vi "Keithley Temperature measurement improved.vi"() -> ()   [LabVIEW 2016]
doc: "This example VI shows how to use thermocouples to take a temperature measurement.\n\nNote:\nFor front panel measurements, make sure the Input switch is in the out position(F)\nFor plug-in card measurements, make sure the Input switch is in the in poisition(R)"
uses:
  Documents/keithley_27xx/Keithley 27XX/Public/Configure/Measurement Specific/Configure FRTD.vi
  Documents/keithley_27xx/Keithley 27XX/Public/Configure/Measurement Specific/Configure Thermocouple.vi
  Documents/keithley_27xx/Keithley 27XX/Public/Configure/Measurement Specific/Configure Thermistor.vi
  Documents/keithley_27xx/Keithley 27XX/Public/Data/Read Multiple Direct.vi
  Documents/keithley_27xx/Keithley 27XX/Keithley 27XX.lvlib
panel:
  in  "Sample Size":dbl
  in  "Sensor Type":string(combo)
  in  "Delta3":dbl=1.0
  in  "Beta3":dbl=0.1
  in  "Alpha3":dbl=0.0038
  in  "Delta2":dbl=1.0
  in  "Beta2":dbl=0.1
  in  "Alpha2":dbl=0.0038
  in  "Delta1":dbl=1.0
  in  "Beta1":dbl=0.1
  in  "Alpha1":dbl=0.0038
  in  "Serial Configuration":T1={"Baud Rate (9600)"=9600, "Flow Control (1: XON/XOFF)"=1, "Termination Char (0:CR)"=0} {"Termination Char (0:CR)" items=["CR", "LF", "CRLF (Do not use)", "LFCR (Do not use)"]; "Flow Control (1: XON/XOFF)" items=["None", "XON/XOFF", "RTS/CTS (2701 Only)", "XON/XOFF & RTS/CTS (2701 Only)"]; "Baud Rate (9600)" items=["300"=300, "600"=600, "1200"=1200, "2400"=2400, "4800"=4800, "9600"=9600, "19.2k"=19200, "38.4k (2701 Only)"=38400, "57.6k (2701 Only)"=57600, "115.2k (2701 Only)"=115200]}
  in  "VISA resource name":refnum<visa-resource-name>="TCPIP0::192.168.69.200::1394::SOCKET"
  out "Output3":dbl[](array[numeric])
  in  "Channel (101) 3":string="117"
  out "Output2":dbl[](array[numeric])
  in  "Channel (101) 2":string="114"
  in  "stop":bool
  out "Output1":dbl[](array[numeric])
  in  "Channel (101)":string="113"
  in  "Temperature (0: Celsius)":u16(ring) items=["Celsius", "Fahrenheit", "Kelvin"]
  # "*For front panel measurements, make sure the Input switch is in the out position(F)*\n  For plug-in card measurements, make sure the Input switch is in the in position(R)"
  # "© 2005 National Instruments Corporation.  ALL RIGHTS RESERVED."
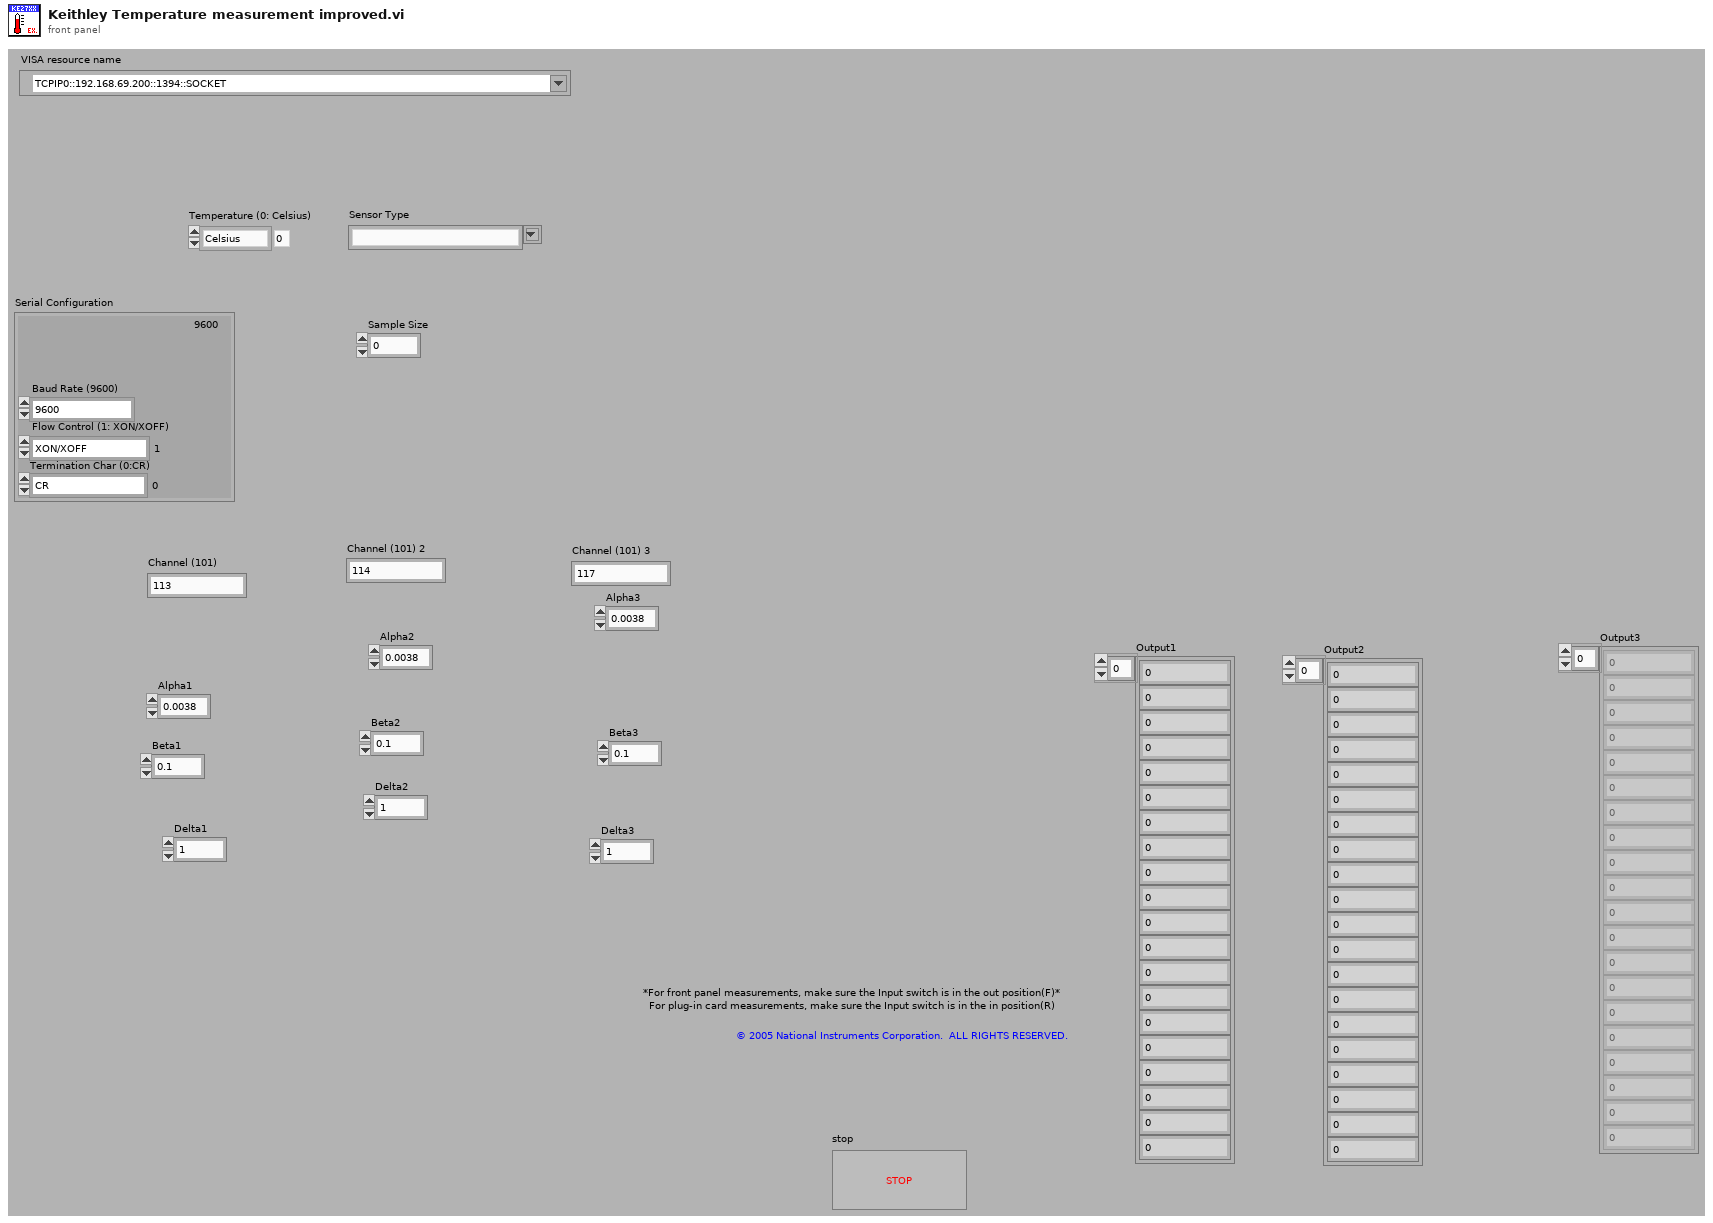
[diagram p1: front panel]
types:
  T1 = cluster{"Baud Rate (9600)":u32, "Flow Control (1: XON/XOFF)":u16, "Termination Char (0:CR)":u16}
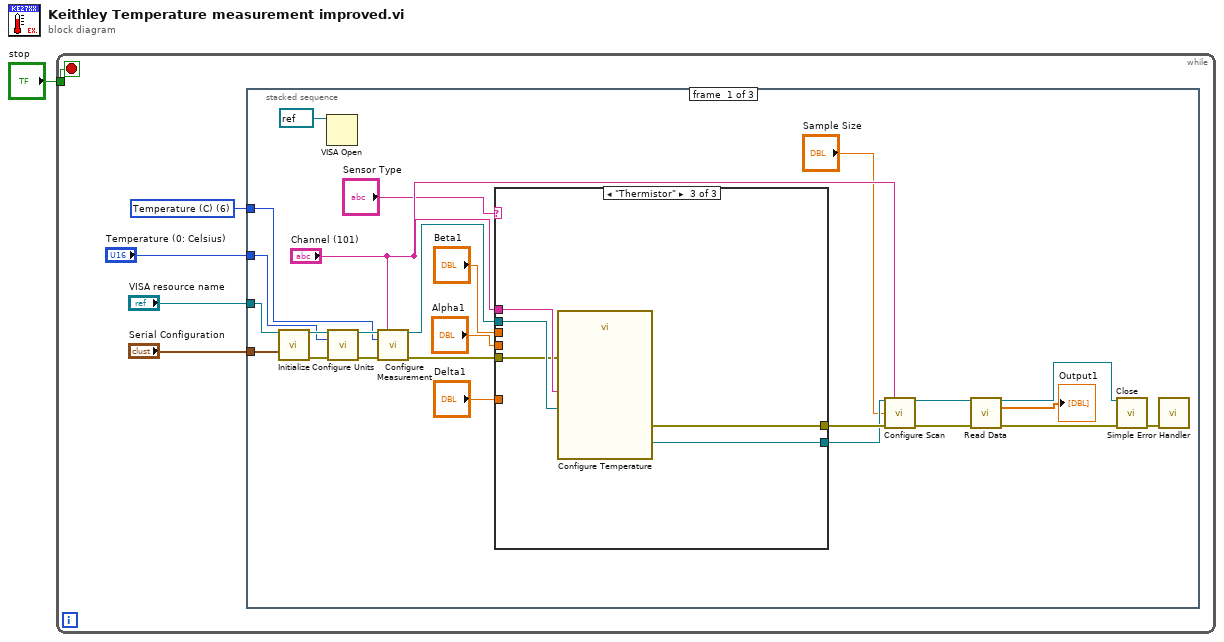
[diagram p0: block diagram]
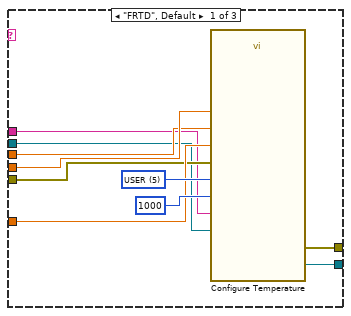
[diagram p2: hidden frame]
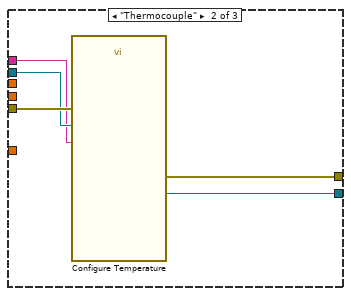
[diagram p3: hidden frame]
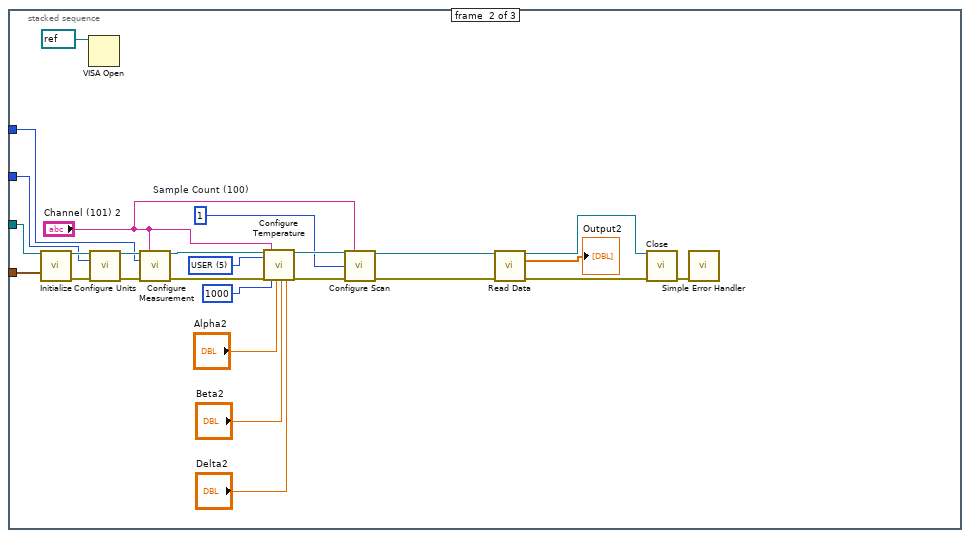
[diagram p4: hidden frame]
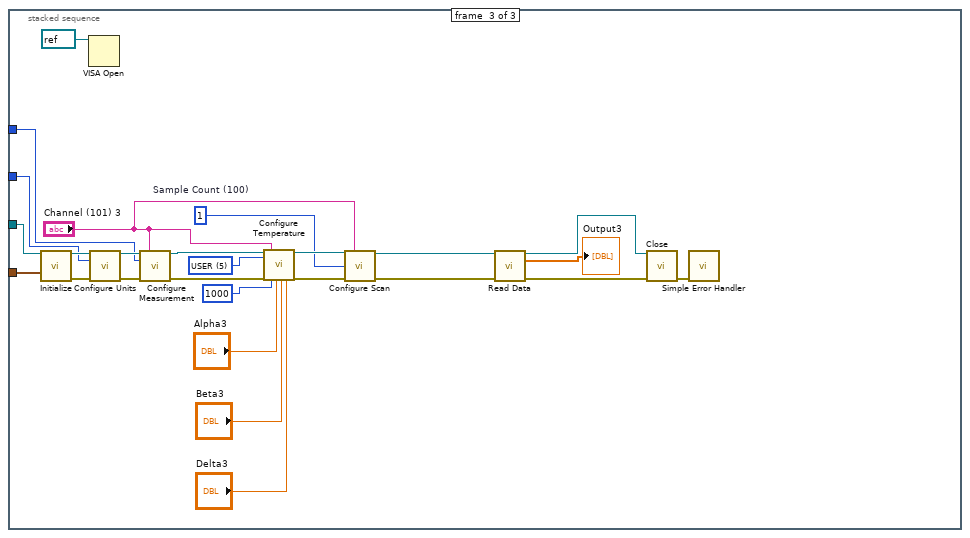
[diagram p5: hidden frame]
diagram:
  n1 = while {
    tunnel: "stop" -> [w2]
    stop <- w2 stop-if-true
    w4 = u16 6 items=["DC Voltage", "AC Voltage", "DC Current", "AC Current", "Resistance", "Four-Wire Resistance", "Temperature (C)", "Frequency", "Period", "Continuity"] ("Function (0: DC Voltage)")
    n2 = stacked-sequence {
      tunnel: "VISA resource name" -> [w20 w57 w84]
      tunnel: "Serial Configuration" -> [w19 w58 w83]
      tunnel: w4 -> [w18 w53 w79]
      tunnel: "Temperature (0: Celsius)" -> [w17 w52 w78]
      frame #0 {
        n3 = call "Initialize.vi"("VISA resource name"=w20, "Serial Configuration"=w19) -> ("VISA resource name out"=w30:refnum<visa-resource-name>, "error out"=w24:errorcluster)  [unwired: 12 in]
        n4 = VISA Open(VISA resource name=refnum<visa-resource-name> refnum) -> ()  [unwired: 4 in, 2 out]
        n5 = call "Configure Units.vi"("VISA resource name"=w30, "Temperature (0: Celsius)"=w17, "error in (no error)"=w24) -> ("VISA resource name out"=w31:refnum<visa-resource-name>, "error out"=w23:errorcluster)  [unwired: 11 in]
        n6 = call "Configure Measurement.vi"("VISA resource name"=w31, "Scan List (Empty)"="Channel (101)", "Function (0: DC Voltage)"=w18, "error in (no error)"=w23) -> ("VISA resource name out"=w10:refnum<visa-resource-name>, "error out"=w11:errorcluster)  [unwired: 10 in]
        n7 = case shown="\"Thermistor\"" "Sensor Type" {
          tunnel: [w40 w45 w51] -> w16
          tunnel: [w41 w46 w50] -> w15
          tunnel: "Delta1" -> [w35 _ _]
          tunnel: "Beta1" -> [w36 _ _]
          tunnel: "Alpha1" -> [w37 _ _]
          tunnel: w11 -> [w34 w44 w47]
          tunnel: w10 -> [w33 w43 w48]
          tunnel: "Channel (101)" -> [w32 w42 w49]
          frame "FRTD", Default {
            w39 = u16 5 items=["PT100", "D100", "F100", "PT3916", "PT385", "USER"] ("FRTD Type (0: PT100)")
            n8 = call-poly "Configure Temperature.vi"("VISA resource name"=w33, "FRTD Type (0: PT100)"=w39, "error in (no error)"=w34, "Scan List (Empty)"=w32, "R Zero (100)"=1000, "Alpha (0.00385)"=w37, "Beta (0.111)"=w36, "Delta (1.507)"=w35) -> ("VISA resource name out"=w41:refnum<visa-resource-name>, "error out"=w40:errorcluster)  [unwired: 10 in]
          }
          frame "Thermocouple" {
            n9 = call-poly "Configure Temperature.vi"("VISA resource name"=w43, "error in (no error)"=w44, "Scan List (Empty)"=w42) -> ("VISA resource name out"=w46:refnum<visa-resource-name>, "error out"=w45:errorcluster)  [unwired: 15 in]
          }
          frame "Thermistor" {
            n10 = call-poly "Configure Temperature.vi"("VISA resource name"=w48, "error in (no error)"=w47, "Scan List (Empty)"=w49) -> ("VISA resource name out"=w50:refnum<visa-resource-name>, "error out"=w51:errorcluster)  [unwired: 15 in]
          }
        }
        n11 = call "Configure Scan.vi"("VISA resource name"=w15, "Channel List (101:110)"="Channel (101)", "Sample Count (100)"="Sample Size", "error in (no error)"=w16) -> ("VISA resource name out"=w27:refnum<visa-resource-name>, "error out"=w28:errorcluster)  [unwired: 10 in]
        n12 = call-poly "Read Data.vi"("VISA resource name"=w27, "error in (no error)"=w28) -> ("VISA resource name out"=w25:refnum<visa-resource-name>, "Measurement Data"=→"Output1":dbl[], "error out"=w26:errorcluster)  [unwired: 8 in, 3 out]
        n13 = call "Close.vi"("VISA resource name"=w25, "error in (no error)"=w26) -> ("error out"=w29:errorcluster)  [unwired: 13 in]
        n14 = call <vilib>:"Simple Error Handler.vi"("error in (no error)"=w29) -> ()  [unwired: 4 in, 5 out]
      }
      frame #1 {
        w62 = u16 5 items=["PT100", "D100", "F100", "PT3916", "PT385", "USER"] ("FRTD Type (0: PT100)")
        w64 = 1  # Sample Count (100)
        n15 = call "Initialize.vi"("VISA resource name"=w57, "Serial Configuration"=w58) -> ("VISA resource name out"=w75:refnum<visa-resource-name>, "error out"=w67:errorcluster)  [unwired: 12 in]
        n16 = VISA Open(VISA resource name=refnum<visa-resource-name> refnum) -> ()  [unwired: 4 in, 2 out]
        n17 = call "Configure Units.vi"("VISA resource name"=w75, "Temperature (0: Celsius)"=w52, "error in (no error)"=w67) -> ("VISA resource name out"=w76:refnum<visa-resource-name>, "error out"=w66:errorcluster)  [unwired: 11 in]
        n18 = call "Configure Measurement.vi"("VISA resource name"=w76, "Scan List (Empty)"="Channel (101) 2", "Function (0: DC Voltage)"=w53, "error in (no error)"=w66) -> ("VISA resource name out"=w65:refnum<visa-resource-name>, "error out"=w77:errorcluster)  [unwired: 10 in]
        n19 = call-poly "Configure Temperature.vi"("VISA resource name"=w65, "FRTD Type (0: PT100)"=w62, "error in (no error)"=w77, "Scan List (Empty)"="Channel (101) 2", "R Zero (100)"=1000, "Alpha (0.00385)"="Alpha2", "Beta (0.111)"="Beta2", "Delta (1.507)"="Delta2") -> ("VISA resource name out"=w73:refnum<visa-resource-name>, "error out"=w72:errorcluster)  [unwired: 10 in]
        n20 = call "Configure Scan.vi"("VISA resource name"=w73, "Channel List (101:110)"="Channel (101) 2", "Sample Count (100)"=w64, "error in (no error)"=w72) -> ("VISA resource name out"=w70:refnum<visa-resource-name>, "error out"=w71:errorcluster)  [unwired: 10 in]
        n21 = call-poly "Read Data.vi"("VISA resource name"=w70, "error in (no error)"=w71) -> ("VISA resource name out"=w68:refnum<visa-resource-name>, "Measurement Data"=→"Output2":dbl[], "error out"=w69:errorcluster)  [unwired: 8 in, 3 out]
        n22 = call "Close.vi"("VISA resource name"=w68, "error in (no error)"=w69) -> ("error out"=w74:errorcluster)  [unwired: 13 in]
        n23 = call <vilib>:"Simple Error Handler.vi"("error in (no error)"=w74) -> ()  [unwired: 4 in, 5 out]
      }
      frame #2 {
        w88 = u16 5 items=["PT100", "D100", "F100", "PT3916", "PT385", "USER"] ("FRTD Type (0: PT100)")
        w90 = 1  # Sample Count (100)
        n24 = call "Initialize.vi"("VISA resource name"=w84, "Serial Configuration"=w83) -> ("VISA resource name out"=w101:refnum<visa-resource-name>, "error out"=w93:errorcluster)  [unwired: 12 in]
        n25 = VISA Open(VISA resource name=refnum<visa-resource-name> refnum) -> ()  [unwired: 4 in, 2 out]
        n26 = call "Configure Units.vi"("VISA resource name"=w101, "Temperature (0: Celsius)"=w78, "error in (no error)"=w93) -> ("VISA resource name out"=w102:refnum<visa-resource-name>, "error out"=w92:errorcluster)  [unwired: 11 in]
        n27 = call "Configure Measurement.vi"("VISA resource name"=w102, "Scan List (Empty)"="Channel (101) 3", "Function (0: DC Voltage)"=w79, "error in (no error)"=w92) -> ("VISA resource name out"=w91:refnum<visa-resource-name>, "error out"=w103:errorcluster)  [unwired: 10 in]
        n28 = call-poly "Configure Temperature.vi"("VISA resource name"=w91, "FRTD Type (0: PT100)"=w88, "error in (no error)"=w103, "Scan List (Empty)"="Channel (101) 3", "R Zero (100)"=1000, "Alpha (0.00385)"="Alpha3", "Beta (0.111)"="Beta3", "Delta (1.507)"="Delta3") -> ("VISA resource name out"=w99:refnum<visa-resource-name>, "error out"=w98:errorcluster)  [unwired: 10 in]
        n29 = call "Configure Scan.vi"("VISA resource name"=w99, "Channel List (101:110)"="Channel (101) 3", "Sample Count (100)"=w90, "error in (no error)"=w98) -> ("VISA resource name out"=w96:refnum<visa-resource-name>, "error out"=w97:errorcluster)  [unwired: 10 in]
        n30 = call-poly "Read Data.vi"("VISA resource name"=w96, "error in (no error)"=w97) -> ("VISA resource name out"=w94:refnum<visa-resource-name>, "Measurement Data"=→"Output3":dbl[], "error out"=w95:errorcluster)  [unwired: 8 in, 3 out]
        n31 = call "Close.vi"("VISA resource name"=w94, "error in (no error)"=w95) -> ("error out"=w100:errorcluster)  [unwired: 13 in]
        n32 = call <vilib>:"Simple Error Handler.vi"("error in (no error)"=w100) -> ()  [unwired: 4 in, 5 out]
      }
    }
  }
